vi "Output.vi"(8 "error in (no error)":errorcluster, 9 "Data Queue":refnum<queue>, 10 "Data Notifier":refnum<notifier>, 11 "Hardware Configuration In":T1={"Task ID"=0, "Volume"=0.0, "Data"={"SignalType"=enum."SineWave", "WhiteNoiseSettings"={"Generate New Data"=FALSE, "Save"=FALSE, "Filter"=TRUE, "Gain"=0}, "SineWaveSttings"={"Frequency"=0.0, "Amplitude"=0.0}}, "Generated Data"={"t0"=timestamp(0 s since 1904-01-01), "dt"=1.0, "Y"=[]}} {"task ID out" format="%.0x"}) -> (0 "error out":errorcluster, 3 "Hardware Configuration Out":T1={"Task ID"=0, "Volume"=0.0, "Data"={"SignalType"=enum."SineWave", "WhiteNoiseSettings"={"Generate New Data"=FALSE, "Save"=FALSE, "Filter"=TRUE, "Gain"=0}, "SineWaveSttings"={"Frequency"=0.0, "Amplitude"=0.0}}, "Generated Data"={"t0"=timestamp(0 s since 1904-01-01), "dt"=1.0, "Y"=[]}} {"task ID out" format="%.0x"})   [LabVIEW 2022 SP3]
doc: "Perform the acquisition. Replace the contents of this diagram with calls to acquisition hardware."
uses:
  Logging/QueuedLoggedData.ctl
  FFT-Data.ctl
  Output Hardware Configuration.ctl
  <vilib>/sound2/lvsound2.llb/Sound Output Task ID.ctl
  Data.ctl
  WhiteNoiseSettings.ctl
  SineWaveSettings.ctl
  <vilib>/sound2/lvsound2.llb/Sound Output Write (DBL Single).vi
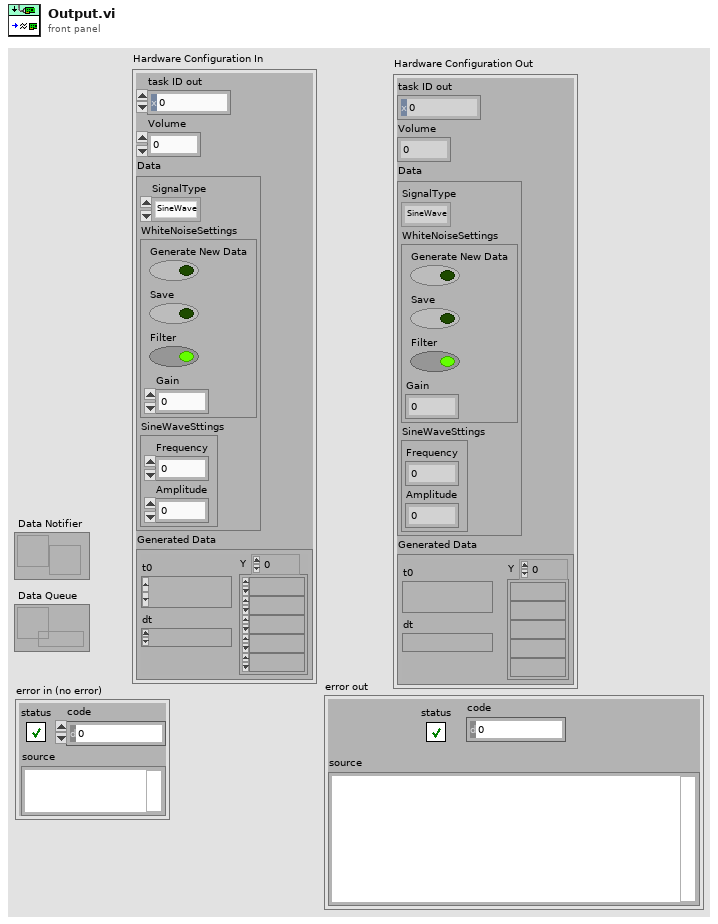
[diagram p1: front panel]
types:
  T1 = typedef "Output Hardware Configuration.ctl" = cluster{"Task ID":T2, "Volume":dbl, "Data":T3, "Generated Data":waveform(dbl)}
  T2 = typedef "Sound Output Task ID.ctl" = u32
  T3 = typedef "Data.ctl" = cluster{"SignalType":enum16{"WhiteNoise", "SineWave"}, "WhiteNoiseSettings":T4, "SineWaveSttings":T5}
  T4 = typedef "WhiteNoiseSettings.ctl" = cluster{"Generate New Data":bool, "Save":bool, "Filter":bool, "Gain":i32}
  T5 = typedef "SineWaveSettings.ctl" = cluster{"Frequency":dbl, "Amplitude":dbl}
  T6 = typedef "QueuedLoggedData.ctl" = cluster{"RawData":waveform(dbl)[], "FFT ":T7[], "Output Data":waveform(dbl)}
  T7 = typedef "FFT-Data.ctl" = cluster{"FFT-Mag":cluster{"t0":dbl, "dt":dbl, "Y":dbl[]}, "FFT-Phase":cluster{"t0":dbl, "dt":dbl, "Y":dbl[]}}
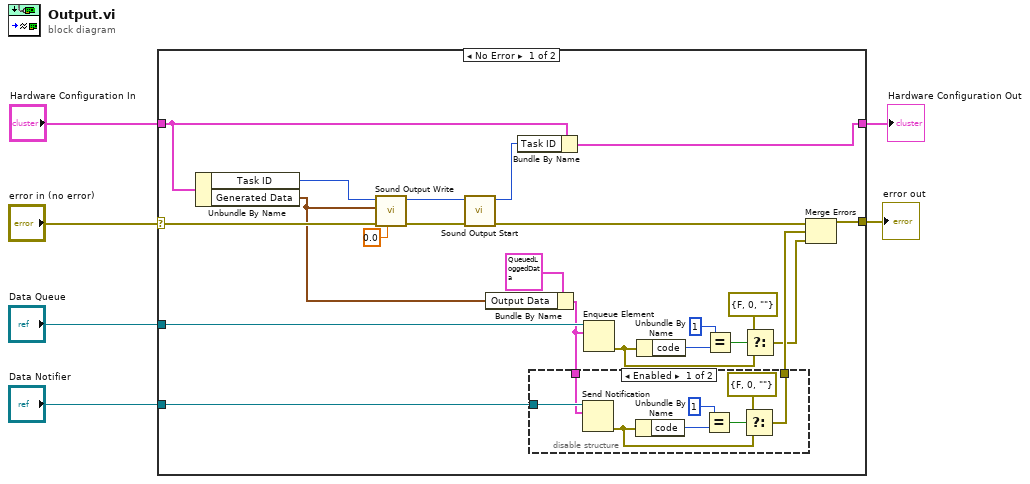
[diagram p0: block diagram]
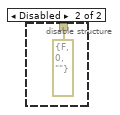
[diagram p2: hidden frame]
diagram:
  n1 = case shown="No Error" "error in (no error)" {
    selector: "error in (no error)" -> [w13 w37]
    tunnel: [w27 w37] -> w5
    tunnel: "Hardware Configuration In" -> [w14 w38]
    tunnel: [w24 w38] -> w1
    tunnel: "Data Notifier" -> [w26 _]
    tunnel: "Data Queue" -> [w25 _]
    frame No Error {
      n2 = Unbundle By Name(w14) -> ("Task ID"=w12:T2, "Generated Data"=w8:waveform(dbl))
      n3 = call-poly <vilib>:"Sound Output Write.vi"("timeout (sec)"=0.0, "data"=w8, "task ID"=w12) -> ("task ID out"=w9:T2)  [unwired: 7 in, 1 out]
      n4 = call <vilib>:"Sound Output Start.vi"("error in (no error)"=w13, "task ID"=w9) -> ("error out"=w10:errorcluster, "task ID out"=w11:T2)  [unwired: 8 in]
      n5 = Bundle By Name(cluster=T6 {"RawData"=[], "FFT "=[], "Output Data"={"t0"=timestamp(0 s since 1904-01-01), "dt"=1.0, "Y"=[]}} ("Cluster"), "Output Data"=w8) -> (w15:T6)
      n6 = Bundle By Name(cluster=w14, "Task ID"=w11) -> (w24:T1)
      n7 = disable-structure shown="Enabled" {
        disable-tunnel: w26 -> [w35 _]
        disable-tunnel: [w34 errorcluster {"status"=FALSE, "code"=0, "source"=""} ("error out")] -> w23
        disable-tunnel: w15 -> [w33 _]
        frame Enabled {
          n8 = Send Notification(notification=w33, notifier=w35) -> (error out=w29:errorcluster)  [unwired: 1 in, 1 out]
          n9 = Unbundle By Name(w29) -> ("code"=w32:i32)
          n10 = Equal?(x=1, y=w32) -> (x = y?=w30:bool)
          n11 = Select(t=errorcluster {"status"=FALSE, "code"=0, "source"=""} ("error constant"), s=w30, f=w29) -> (s? t:f=w34:errorcluster)
        }
        frame Disabled {
        }
      }
      n12 = Enqueue Element(queue=w25, element=w15) -> (error out=w21:errorcluster)  [unwired: 2 in, 2 out]
      n13 = Unbundle By Name(w21) -> ("code"=w18:i32)
      n14 = Equal?(x=1, y=w18) -> (x = y?=w20:bool)
      n15 = Select(t=errorcluster {"status"=FALSE, "code"=0, "source"=""} ("error constant"), s=w20, f=w21) -> (s? t:f=w17:errorcluster)
      n16 = Merge Errors(w10, w23, w17) -> (w27:errorcluster)
    }
    frame Error {
    }
  }
  "error out" <- w5
  "Hardware Configuration Out" <- w1
